vi "Create Evaluations.vi"(8 "error in (no error)":errorcluster, 11 "IEvaluation in":refnum<class "Servo Gain.lvclass">) -> (0 "error out":errorcluster, 2 "Evaluations Out":T1[](array[typedef]) {"Low Limit" format="%#_13g"; "SI Scaling" items=["femto"=-15, "pico"=-12, "nano"=-9, "micro"=-6, "milli"=-3, "percent"=-2, ""=0, "kilo"=3, "mega"=6, "giga"=9, "tera"=12]}, 3 "IEvaluation out":refnum<class "Servo Gain.lvclass">)   [LabVIEW 2016, in "SeqAuto Evaluations.lvlib" / "Servo Gain.lvclass"]
uses:
  Servo Gain.lvclass
  C:/Sequence Automation/Plugins/SeqAuto IEvaluation.lvlibp/SeqAuto IEvaluation.lvclass
  Plugins/TestStand API Tools (TSAT).lvlibp/Evaluation Actions/Includes/Controls/TSAT Evaluation.ctl
  Plugins/TestStand API Tools (TSAT).lvlibp/Evaluation Actions/Includes/Controls/TSAT Eval SI Unit Scaling.ctl
  Plugins/TestStand API Tools (TSAT).lvlibp/Evaluation Actions/Includes/Controls/TSAT Evaluation Type.ctl
  Servo Gain.lvclass/Servo Gain.ctl
  Plugins/SeqAuto IEvaluation.lvlibp/Read Measurement Name.vi
  Plugins/TestStand API Tools (TSAT).lvlibp/Evaluation Actions/TSAT Evaluation Actions.lvlib
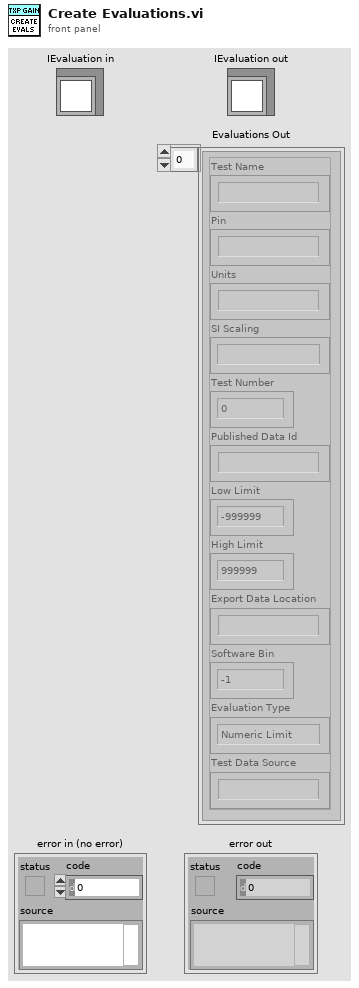
[diagram p1: front panel]
types:
  T1 = typedef "TestStand API Tools (TSAT).lvlibp/TSAT Evaluation Actions.lvlib/TSAT Evaluation.ctl" = cluster{"Test Name":string, "Pin":string, "Units":string, "SI Scaling":T2, "Test Number":i32, "Published Data Id":string, "Low Limit":dbl, "High Limit":dbl, "Export Data Location":string, "Software Bin":i64, "Evaluation Type":T3, "Test Data Source":string}
  T2 = typedef "TestStand API Tools (TSAT).lvlibp/TSAT Evaluation Actions.lvlib/TSAT Eval SI Unit Scaling.ctl" = i16
  T3 = typedef "TestStand API Tools (TSAT).lvlibp/TSAT Evaluation Actions.lvlib/TSAT Evaluation Type.ctl" = enum16{"Numeric Limit", "Pass/Fail", "None"}
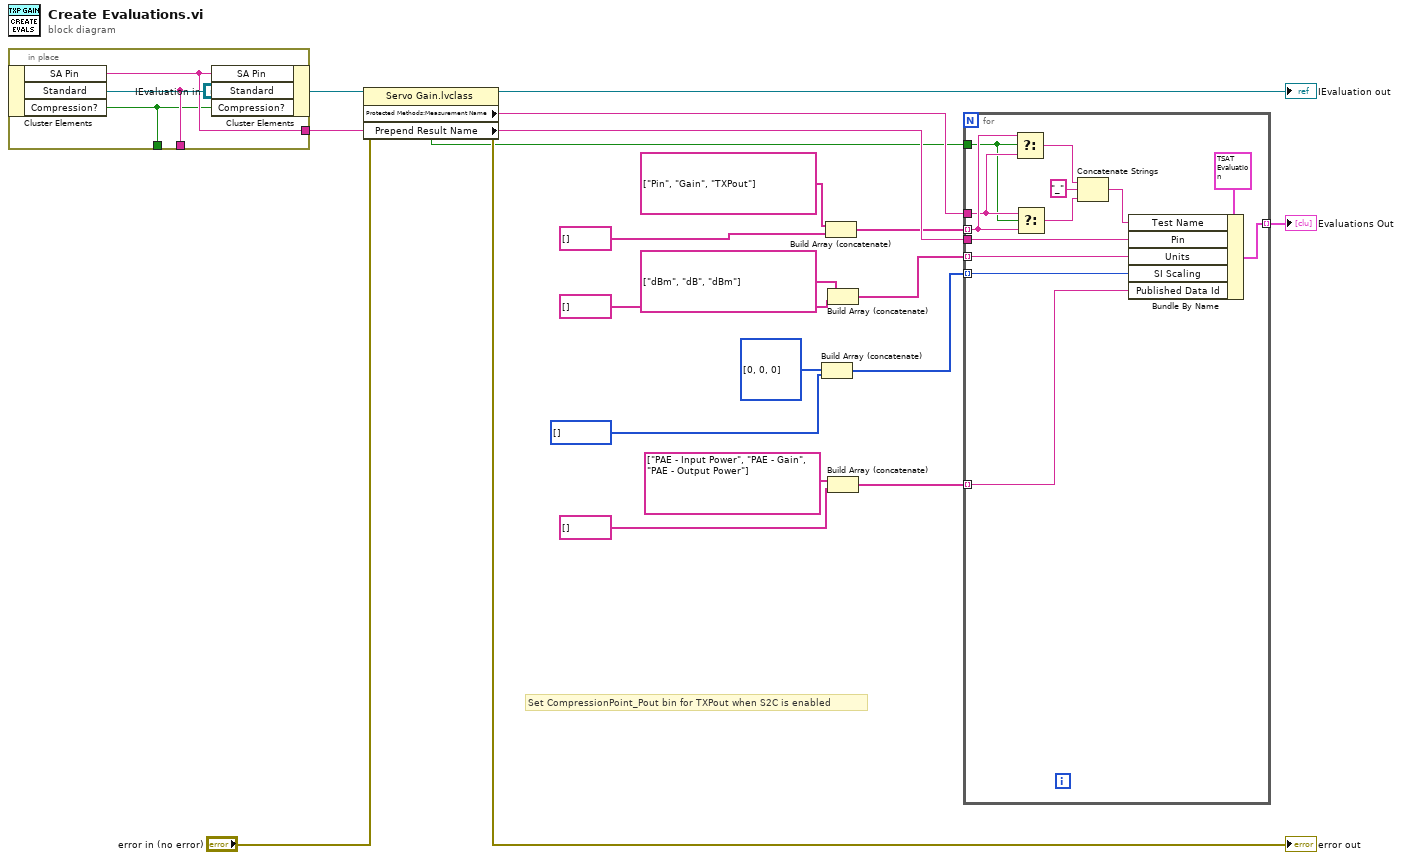
[diagram p0: block diagram]
diagram:
  w9 = T2[] [] items=["femto"=-15, "pico"=-12, "nano"=-9, "micro"=-6, "milli"=-3, "percent"=-2, ""=0, "kilo"=3, "mega"=6, "giga"=9, "tera"=12]
  w8 = T2[] [0, 0, 0] items=["femto"=-15, "pico"=-12, "nano"=-9, "micro"=-6, "milli"=-3, "percent"=-2, ""=0, "kilo"=3, "mega"=6, "giga"=9, "tera"=12]
  # "Set CompressionPoint_Pout bin for TXPout when S2C is enabled"
  n1 = in-place {
    in-place-border: [w24] -> w18
    in-place-border: [w23] -> _
    in-place-border: [w22] -> _
    n2 = in-place-cluster #1("IEvaluation in") -> ("SA Pin"=w24:string, "Standard"=w23:string, "Compression?"=w22:bool)
    n3 = in-place-cluster #1("SA Pin"=w24, "Standard"=w23, "Compression?"=w22) -> (w14:refnum<class "Servo Gain.lvclass">)
  }
  n4 = property class="Servo Gain.lvclass"(reference=w14, error in="error in (no error)") -> (reference out=→"IEvaluation out":refnum<class "Servo Gain.lvclass">, error out=→"error out":errorcluster, "Protected Methods:Measurement Name"=w2:string, "Prepend Result Name"=w1:bool)
  n5 = Build Array (concatenate)(w8, w9) -> (w7:T2[])
  n6 = Build Array (concatenate)(string[] ["Pin", "Gain", "TXPout"], string[] []) -> (w12:string[])
  n7 = Build Array (concatenate)(string[] ["dBm", "dB", "dBm"], string[] []) -> (w6:string[])
  n8 = Build Array (concatenate)(string[] ["PAE - Input Power", "PAE - Gain", "PAE - Output Power"], string[] []) -> (w3:string[])
  n9 = for {
    tunnel: [w36] -> w20 mode=indexing
    tunnel: w18 -> [w35]
    tunnel: w2 -> [w26]
    tunnel: w12 -> [w27] mode=indexing
    tunnel: w7 -> [w33] mode=indexing
    tunnel: w6 -> [w32] mode=indexing
    tunnel: w3 -> [w31] mode=indexing
    tunnel: w1 -> [w25]
    n10 = Select(t=w27, s=w25, f=w26) -> (s? t:f=w28:string)
    n11 = Select(t=w26, s=w25, f=w27) -> (s? t:f=w29:string)
    n12 = Concatenate Strings(w28, "_" ("string"), w29) -> (w34:string)
    n13 = Bundle By Name(cluster=T1 {"Test Name"="", "Pin"="", "Units"="", "SI Scaling"=0, "Test Number"=0, "Published Data Id"="", "Low Limit"=-999999.0, "High Limit"=999999.0, "Export Data Location"="", "Software Bin"=-1, "Evaluation Type"=enum."Numeric Limit", "Test Data Source"=""} ("Evaluation"), "Test Name"=w34, "Pin"=w35, "Units"=w32, "SI Scaling"=w33, "Published Data Id"=w31) -> (w36:T1)
  }
  "Evaluations Out" <- w20
